vi "Read Menu Reference.vi"(8 "error in (no error)":errorcluster, 11 "Front Panel Menu in":refnum<class "Front Panel Menu.lvclass">) -> (0 "error out":errorcluster, 2 "Menu Reference":refnum<k9>, 3 "Front Panel Menu out":refnum<class "Front Panel Menu.lvclass">)   [LabVIEW 2024, in "Front Panel Menu.lvclass"]
uses:
  Front Panel Menu.lvclass
  Front Panel Menu.lvclass/Front Panel Menu.ctl
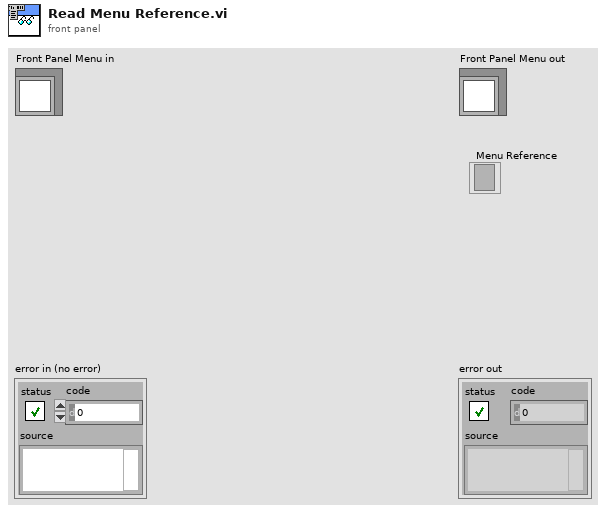
[diagram p1: front panel]
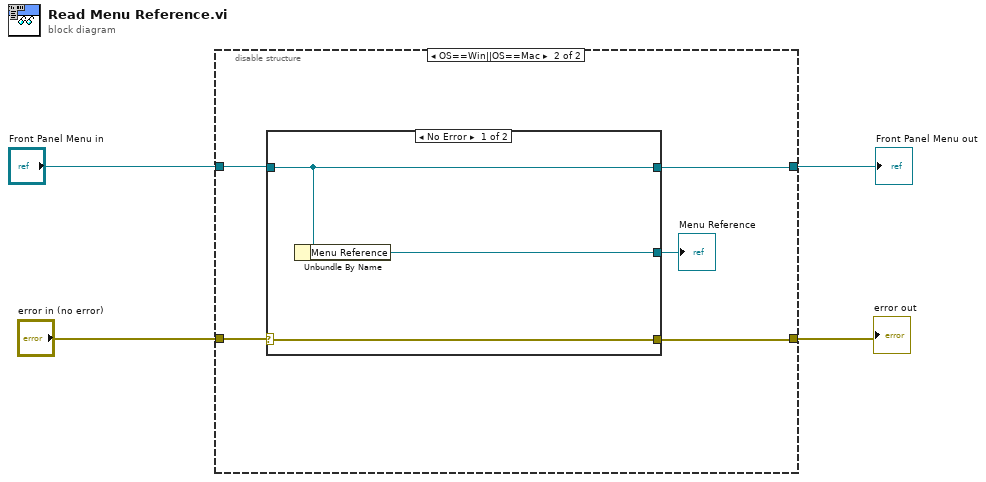
[diagram p0: block diagram]
diagram:
  n1 = disable-structure shown="OS==Win||OS==Mac" {
    disable-tunnel: "Front Panel Menu in" -> [w6 w10]
    disable-tunnel: [w6 w8] -> w3
    disable-tunnel: "error in (no error)" -> [w5 w9]
    disable-tunnel: [w5 w7] -> w1
    frame condition #0 {
    }
    frame condition #1 (active) {
      n2 = case shown="No Error" w9 {
        selector: w9 -> [w14 w15]
        tunnel: [w14 w15] -> w7
        tunnel: [w13 w16] -> w8
        tunnel: w10 -> [w13 w16]
        tunnel: [w12 _] -> w11
        frame No Error {
          n3 = Unbundle By Name(w13) -> ("Menu Reference"=w12:refnum<k9>)
        }
        frame Error {
        }
      }
      "Menu Reference" <- w11
    }
  }
  "Front Panel Menu out" <- w3
  "error out" <- w1
